vi "Acquisition and Generation Engine.vi"() -> ()   [LabVIEW 2015]
uses:
  Controls/Wave Generator Control.ctl
  Controls/WT1800 Readings.ctl
  Controls/WT1800 Measurements.ctl
  Controls/DSA Readings.ctl
  Controls/DSA Measurements.ctl
  Controls/WT1800 Functions.ctl
  Controls/DSA Functions.ctl
  Controls/Settings Control.ctl
  Controls/Channel Configuration Cluster.ctl
  Controls/Channel Configuration List.ctl
  Controls/Gain Averages.ctl
  Controls/Channel Configuration Cluster High Current.ctl
  Controls/Gain Array.ctl
panel:
  out "Supply Low":bool
  out "Test Time":dbl format="%<%H:%M:%S>t"
  in  "Tab Control":enum32{"Numeric", "Graph", "GUI Controls"}(tab)
  out "DSA Measurements":T1 {"Vrms" format="%.3f"; "Vdc" format="%.3f"; "Vpk+" format="%.3f"; "Vpk-" format="%.3f"; "Vpkpk" format="%.3f"}
  out "WT1800 Measurements":T3 {"Vrms" format="%.3f"; "Irms" format="%.3f"; "Power" format="%.3f"; "Vpkpk" format="%.3f"; "Ipkpk" format="%.3f"}
  out "DSA Averages":T1 {"Vrms" format="%.3f"; "Vdc" format="%.3f"; "Vpk+" format="%.3f"; "Vpk-" format="%.3f"; "Vpkpk" format="%.3f"}
  out "WT1800 Functions":T5
  out "WT1800 Averages":T3 {"Vrms" format="%.3f"; "Irms" format="%.3f"; "Power" format="%.3f"; "Vpkpk" format="%.3f"; "Ipkpk" format="%.3f"}
  out "DSA Functions":T6
  out "Graph":dbl[][](graph)
  in  "Wave Generator Cluster":T7={"Signal Amplitude [Vrms]"=0.1, "Signal Type"=0, "Frequency Range [Hz]"={"start"=150.0, "stop"=0.0}, "Waveform Duration [Seconds]"=10.0} {"Signal Type" items=["Sine", "Linear Chirp", "Log Chirp", "Pink Noise", "Periodic Random Noise", "Uniform White Noise", "Gaussian White Noise", "11db4816 Wave File"]}
  in  "Settings Cluster":T8={"Supply Voltage [Vdc]"=14.4, "Max Supply Current [Idc]"=50.0, "Settling Delay"=10.0, "Temp Criteria"=0.0, "Voltage Steps [Vrms]"=[0.25, 0.5, 1.0, 1.95, 3.0, 3.9, 5.5], "User Notes"="", "Config Wave File Path"=path "", "Config Voltage [Vrms]"=0.0, "Channel Configuration List"={"Channel Configuration Cluster"={"Input"=enum."---", "Enable"=FALSE, "User Notes"="", "Voltage Range"=15.0, "Current Range"=2.5}, "Channel Configuration Cluster 2"={"Input"=enum."---", "Enable"=FALSE, "User Notes"="", "Voltage Range"=15.0, "Current Range"=2.5}, "Channel Configuration Cluster 3"={"Input"=enum."---", "Enable"=FALSE, "User Notes"="", "Voltage Range"=15.0, "Current Range"=2.5}, "Channel Configuration Cluster 4"={"Input"=enum."---", "Enable"=FALSE, "User Notes"="", "Voltage Range"=15.0, "Current Range"=2.5}, "Channel Configuration Cluster 5"={"Input"=enum."---", "Enable"=FALSE, "User Notes"="", "Voltage Range"=15.0, "Current Range"=2.5}, "Channel Configuration Cluster 6"={"Input"=enum."---", "Enable"=FALSE, "User Notes"="", "Voltage Range"=15.0, "Current Range"=2.5}, "Channel Configuration Cluster 7"={"Input"=enum."---", "Enable"=FALSE, "User Notes"="", "Voltage Range"=15.0, "Current Range"=2.5}, "Channel Configuration Cluster 8"={"Input"=enum."---", "Enable"=FALSE, "User Notes"="", "Voltage Range"=15.0, "Current Range"=2.5}, "Channel Configuration Cluster 9"={"Input"=enum."---", "Enable"=FALSE, "User Notes"="", "Voltage Range"=15.0, "Current Range"=2.5}, "Channel Configuration Cluster 10"={"Input"=enum."---", "Enable"=FALSE, "User Notes"="", "Voltage Range"=15.0, "Current Range"=25.0}, "Channel Configuration Cluster 11"={"Input"=enum."---", "Enable"=FALSE, "User Notes"="", "Voltage Range"=15.0, "Current Range"=25.0}, "Channel Configuration Cluster 12"={"Input"=enum."---", "Enable"=FALSE, "User Notes"="", "Voltage Range"=15.0, "Current Range"=25.0}, "Channel Configuration Cluster 13"={"Input"=enum."---", "Enable"=FALSE, "User Notes"="", "Voltage Range"=15.0, "Current Range"=25.0}, "Channel Configuration Cluster 14"={"Input"=enum."---", "Enable"=FALSE, "User Notes"="", "Voltage Range"=15.0, "Current Range"=25.0}, "Channel Configuration Cluster 15"={"Input"=enum."---", "Enable"=FALSE, "User Notes"="", "Voltage Range"=15.0, "Current Range"=25.0}, "Channel Configuration Cluster 16"={"Input"=enum."---", "Enable"=FALSE, "User Notes"="", "Voltage Range"=15.0, "Current Range"=25.0}, "Channel Configuration Cluster 17"={"Input"=enum."---", "Enable"=FALSE, "User Notes"="", "Voltage Range"=15.0, "Current Range"=25.0}}, "User Gains"={"Gain 1"=0.0, "Gain 2"=0.0, "Gain 3"=0.0, "Gain 4"=0.0, "Gain 5"=0.0, "Gain 6"=0.0}, "Gains"={"Gain 1"=0.0, "Gain 2"=0.0, "Gain 3"=0.0, "Gain 4"=0.0, "Gain 5"=0.0, "Gain 6"=0.0}, "Gain Array"={"Gain 1"=0.0, "Gain 2"=0.0, "Gain 3"=0.0, "Gain 4"=0.0, "Gain 5"=0.0, "Gain 6"=0.0, "Gain 7"=0.0, "Gain 8"=0.0, "Gain 9"=0.0, "Gain 10"=0.0, "Gain 11"=0.0, "Gain 12"=0.0, "Gain 13"=0.0, "Gain 14"=0.0, "Gain 15"=0.0, "Gain 16"=0.0, "Gain 17"=0.0}, "Wave File Path 1"=path "", "Wave File Path 2"=path "", "Wave File Path 3"=path "", "Wave File Path 4"=path "", "Range"=FALSE, "CF"=FALSE} {"Gain Array"."Gain 17" format="%.2f"; "Gain Array"."Gain 16" format="%.2f"; "Gain Array"."Gain 15" format="%.2f"; "Gain Array"."Gain 14" format="%.2f"; "Gain Array"."Gain 13" format="%.2f"; "Gain Array"."Gain 12" format="%.2f"; "Gain Array"."Gain 11" format="%.2f"; "Gain Array"."Gain 10" format="%.2f"; "Gain Array"."Gain 9" format="%.2f"; "Gain Array"."Gain 8" format="%.2f"; "Gain Array"."Gain 7" format="%.2f"; "Gain Array"."Gain 6" format="%.2f"; "Gain Array"."Gain 5" format="%.2f"; "Gain Array"."Gain 4" format="%.2f"; "Gain Array"."Gain 3" format="%.2f"; "Gain Array"."Gain 2" format="%.2f"; "Gain Array"."Gain 1" format="%.2f"; "Gains"."Gain 6" format="%.2f"; "Gains"."Gain 5" format="%.2f"; "Gains"."Gain 4" format="%.2f"; "Gains"."Gain 3" format="%.2f"; "Gains"."Gain 2" format="%.2f"; "Gains"."Gain 1" format="%.2f"; "User Gains"."Gain 6" format="%.2f"; "User Gains"."Gain 5" format="%.2f"; "User Gains"."Gain 4" format="%.2f"; "User Gains"."Gain 3" format="%.2f"; "User Gains"."Gain 2" format="%.2f"; "User Gains"."Gain 1" format="%.2f"; "Channel Configuration List"."Channel Configuration Cluster 17"."Current Range" items=["1 <500m>"=0.5, "2 <1>"=1.0, "5 <2.5>"=2.5, "10 <5>"=5.0, "20 <10>"=10.0, "50 <25>"=25.0]; "Channel Configuration List"."Channel Configuration Cluster 17"."Voltage Range" items=["1.5 <0.75>"=0.75, "3 <1.5>"=1.5, "6 <3>"=3.0, "10 <5>"=5.0, "15 <7.5>"=7.5, "30 <15>"=15.0, "60 <30>"=30.0, "100 <50>"=50.0, "150 <75>"=75.0, "300 <150>"=150.0, "600 <300>"=300.0, "1000 <500>"=500.0]; "Channel Configuration List"."Channel Configuration Cluster 16"."Current Range" items=["1 <500m>"=0.5, "2 <1>"=1.0, "5 <2.5>"=2.5, "10 <5>"=5.0, "20 <10>"=10.0, "50 <25>"=25.0]; "Channel Configuration List"."Channel Configuration Cluster 16"."Voltage Range" items=["1.5 <0.75>"=0.75, "3 <1.5>"=1.5, "6 <3>"=3.0, "10 <5>"=5.0, "15 <7.5>"=7.5, "30 <15>"=15.0, "60 <30>"=30.0, "100 <50>"=50.0, "150 <75>"=75.0, "300 <150>"=150.0, "600 <300>"=300.0, "1000 <500>"=500.0]; "Channel Configuration List"."Channel Configuration Cluster 15"."Current Range" items=["1 <500m>"=0.5, "2 <1>"=1.0, "5 <2.5>"=2.5, "10 <5>"=5.0, "20 <10>"=10.0, "50 <25>"=25.0]; "Channel Configuration List"."Channel Configuration Cluster 15"."Voltage Range" items=["1.5 <0.75>"=0.75, "3 <1.5>"=1.5, "6 <3>"=3.0, "10 <5>"=5.0, "15 <7.5>"=7.5, "30 <15>"=15.0, "60 <30>"=30.0, "100 <50>"=50.0, "150 <75>"=75.0, "300 <150>"=150.0, "600 <300>"=300.0, "1000 <500>"=500.0]; "Channel Configuration List"."Channel Configuration Cluster 14"."Current Range" items=["1 <500m>"=0.5, "2 <1>"=1.0, "5 <2.5>"=2.5, "10 <5>"=5.0, "20 <10>"=10.0, "50 <25>"=25.0]; "Channel Configuration List"."Channel Configuration Cluster 14"."Voltage Range" items=["1.5 <0.75>"=0.75, "3 <1.5>"=1.5, "6 <3>"=3.0, "10 <5>"=5.0, "15 <7.5>"=7.5, "30 <15>"=15.0, "60 <30>"=30.0, "100 <50>"=50.0, "150 <75>"=75.0, "300 <150>"=150.0, "600 <300>"=300.0, "1000 <500>"=500.0]; "Channel Configuration List"."Channel Configuration Cluster 13"."Current Range" items=["1 <500m>"=0.5, "2 <1>"=1.0, "5 <2.5>"=2.5, "10 <5>"=5.0, "20 <10>"=10.0, "50 <25>"=25.0]; "Channel Configuration List"."Channel Configuration Cluster 13"."Voltage Range" items=["1.5 <0.75>"=0.75, "3 <1.5>"=1.5, "6 <3>"=3.0, "10 <5>"=5.0, "15 <7.5>"=7.5, "30 <15>"=15.0, "60 <30>"=30.0, "100 <50>"=50.0, "150 <75>"=75.0, "300 <150>"=150.0, "600 <300>"=300.0, "1000 <500>"=500.0]; "Channel Configuration List"."Channel Configuration Cluster 12"."Current Range" items=["1 <500m>"=0.5, "2 <1>"=1.0, "5 <2.5>"=2.5, "10 <5>"=5.0, "20 <10>"=10.0, "50 <25>"=25.0]; "Channel Configuration List"."Channel Configuration Cluster 12"."Voltage Range" items=["1.5 <0.75>"=0.75, "3 <1.5>"=1.5, "6 <3>"=3.0, "10 <5>"=5.0, "15 <7.5>"=7.5, "30 <15>"=15.0, "60 <30>"=30.0, "100 <50>"=50.0, "150 <75>"=75.0, "300 <150>"=150.0, "600 <300>"=300.0, "1000 <500>"=500.0]; "Channel Configuration List"."Channel Configuration Cluster 11"."Current Range" items=["1 <500m>"=0.5, "2 <1>"=1.0, "5 <2.5>"=2.5, "10 <5>"=5.0, "20 <10>"=10.0, "50 <25>"=25.0]; "Channel Configuration List"."Channel Configuration Cluster 11"."Voltage Range" items=["1.5 <0.75>"=0.75, "3 <1.5>"=1.5, "6 <3>"=3.0, "10 <5>"=5.0, "15 <7.5>"=7.5, "30 <15>"=15.0, "60 <30>"=30.0, "100 <50>"=50.0, "150 <75>"=75.0, "300 <150>"=150.0, "600 <300>"=300.0, "1000 <500>"=500.0]; "Channel Configuration List"."Channel Configuration Cluster 10"."Current Range" items=["1 <500m>"=0.5, "2 <1>"=1.0, "5 <2.5>"=2.5, "10 <5>"=5.0, "20 <10>"=10.0, "50 <25>"=25.0]; "Channel Configuration List"."Channel Configuration Cluster 10"."Voltage Range" items=["1.5 <0.75>"=0.75, "3 <1.5>"=1.5, "6 <3>"=3.0, "10 <5>"=5.0, "15 <7.5>"=7.5, "30 <15>"=15.0, "60 <30>"=30.0, "100 <50>"=50.0, "150 <75>"=75.0, "300 <150>"=150.0, "600 <300>"=300.0, "1000 <500>"=500.0]; "Channel Configuration List"."Channel Configuration Cluster 9"."Voltage Range" items=["1.5 <0.75>"=0.75, "3 <1.5>"=1.5, "6 <3>"=3.0, "10 <5>"=5.0, "15 <7.5>"=7.5, "30 <15>"=15.0, "60 <30>"=30.0, "100 <50>"=50.0, "150 <75>"=75.0, "300 <150>"=150.0, "600 <300>"=300.0, "1000 <500>"=500.0]; "Channel Configuration List"."Channel Configuration Cluster 9"."Current Range" items=["10m <5m>"=0.005, "20m <10m>"=0.01, "50m <25m>"=0.025, "100m <50m>"=0.05, "200m <100m>"=0.1, "500m <250m>"=0.25, "1 <500m>"=0.5, "2 <1>"=1.0, "5 <2.5>"=2.5]; "Channel Configuration List"."Channel Configuration Cluster 8"."Voltage Range" items=["1.5 <0.75>"=0.75, "3 <1.5>"=1.5, "6 <3>"=3.0, "10 <5>"=5.0, "15 <7.5>"=7.5, "30 <15>"=15.0, "60 <30>"=30.0, "100 <50>"=50.0, "150 <75>"=75.0, "300 <150>"=150.0, "600 <300>"=300.0, "1000 <500>"=500.0]; "Channel Configuration List"."Channel Configuration Cluster 8"."Current Range" items=["10m <5m>"=0.005, "20m <10m>"=0.01, "50m <25m>"=0.025, "100m <50m>"=0.05, "200m <100m>"=0.1, "500m <250m>"=0.25, "1 <500m>"=0.5, "2 <1>"=1.0, "5 <2.5>"=2.5]; "Channel Configuration List"."Channel Configuration Cluster 7"."Voltage Range" items=["1.5 <0.75>"=0.75, "3 <1.5>"=1.5, "6 <3>"=3.0, "10 <5>"=5.0, "15 <7.5>"=7.5, "30 <15>"=15.0, "60 <30>"=30.0, "100 <50>"=50.0, "150 <75>"=75.0, "300 <150>"=150.0, "600 <300>"=300.0, "1000 <500>"=500.0]; "Channel Configuration List"."Channel Configuration Cluster 7"."Current Range" items=["10m <5m>"=0.005, "20m <10m>"=0.01, "50m <25m>"=0.025, "100m <50m>"=0.05, "200m <100m>"=0.1, "500m <250m>"=0.25, "1 <500m>"=0.5, "2 <1>"=1.0, "5 <2.5>"=2.5]; "Channel Configuration List"."Channel Configuration Cluster 6"."Voltage Range" items=["1.5 <0.75>"=0.75, "3 <1.5>"=1.5, "6 <3>"=3.0, "10 <5>"=5.0, "15 <7.5>"=7.5, "30 <15>"=15.0, "60 <30>"=30.0, "100 <50>"=50.0, "150 <75>"=75.0, "300 <150>"=150.0, "600 <300>"=300.0, "1000 <500>"=500.0]; "Channel Configuration List"."Channel Configuration Cluster 6"."Current Range" items=["10m <5m>"=0.005, "20m <10m>"=0.01, "50m <25m>"=0.025, "100m <50m>"=0.05, "200m <100m>"=0.1, "500m <250m>"=0.25, "1 <500m>"=0.5, "2 <1>"=1.0, "5 <2.5>"=2.5]; "Channel Configuration List"."Channel Configuration Cluster 5"."Voltage Range" items=["1.5 <0.75>"=0.75, "3 <1.5>"=1.5, "6 <3>"=3.0, "10 <5>"=5.0, "15 <7.5>"=7.5, "30 <15>"=15.0, "60 <30>"=30.0, "100 <50>"=50.0, "150 <75>"=75.0, "300 <150>"=150.0, "600 <300>"=300.0, "1000 <500>"=500.0]; "Channel Configuration List"."Channel Configuration Cluster 5"."Current Range" items=["10m <5m>"=0.005, "20m <10m>"=0.01, "50m <25m>"=0.025, "100m <50m>"=0.05, "200m <100m>"=0.1, "500m <250m>"=0.25, "1 <500m>"=0.5, "2 <1>"=1.0, "5 <2.5>"=2.5]; "Channel Configuration List"."Channel Configuration Cluster 4"."Voltage Range" items=["1.5 <0.75>"=0.75, "3 <1.5>"=1.5, "6 <3>"=3.0, "10 <5>"=5.0, "15 <7.5>"=7.5, "30 <15>"=15.0, "60 <30>"=30.0, "100 <50>"=50.0, "150 <75>"=75.0, "300 <150>"=150.0, "600 <300>"=300.0, "1000 <500>"=500.0]; "Channel Configuration List"."Channel Configuration Cluster 4"."Current Range" items=["10m <5m>"=0.005, "20m <10m>"=0.01, "50m <25m>"=0.025, "100m <50m>"=0.05, "200m <100m>"=0.1, "500m <250m>"=0.25, "1 <500m>"=0.5, "2 <1>"=1.0, "5 <2.5>"=2.5]; "Channel Configuration List"."Channel Configuration Cluster 3"."Voltage Range" items=["1.5 <0.75>"=0.75, "3 <1.5>"=1.5, "6 <3>"=3.0, "10 <5>"=5.0, "15 <7.5>"=7.5, "30 <15>"=15.0, "60 <30>"=30.0, "100 <50>"=50.0, "150 <75>"=75.0, "300 <150>"=150.0, "600 <300>"=300.0, "1000 <500>"=500.0]; "Channel Configuration List"."Channel Configuration Cluster 3"."Current Range" items=["10m <5m>"=0.005, "20m <10m>"=0.01, "50m <25m>"=0.025, "100m <50m>"=0.05, "200m <100m>"=0.1, "500m <250m>"=0.25, "1 <500m>"=0.5, "2 <1>"=1.0, "5 <2.5>"=2.5]; "Channel Configuration List"."Channel Configuration Cluster 2"."Voltage Range" items=["1.5 <0.75>"=0.75, "3 <1.5>"=1.5, "6 <3>"=3.0, "10 <5>"=5.0, "15 <7.5>"=7.5, "30 <15>"=15.0, "60 <30>"=30.0, "100 <50>"=50.0, "150 <75>"=75.0, "300 <150>"=150.0, "600 <300>"=300.0, "1000 <500>"=500.0]; "Channel Configuration List"."Channel Configuration Cluster 2"."Current Range" items=["10m <5m>"=0.005, "20m <10m>"=0.01, "50m <25m>"=0.025, "100m <50m>"=0.05, "200m <100m>"=0.1, "500m <250m>"=0.25, "1 <500m>"=0.5, "2 <1>"=1.0, "5 <2.5>"=2.5]; "Channel Configuration List"."Channel Configuration Cluster"."Voltage Range" items=["1.5 <0.75>"=0.75, "3 <1.5>"=1.5, "6 <3>"=3.0, "10 <5>"=5.0, "15 <7.5>"=7.5, "30 <15>"=15.0, "60 <30>"=30.0, "100 <50>"=50.0, "150 <75>"=75.0, "300 <150>"=150.0, "600 <300>"=300.0, "1000 <500>"=500.0]; "Channel Configuration List"."Channel Configuration Cluster"."Current Range" items=["10m <5m>"=0.005, "20m <10m>"=0.01, "50m <25m>"=0.025, "100m <50m>"=0.05, "200m <100m>"=0.1, "500m <250m>"=0.25, "1 <500m>"=0.5, "2 <1>"=1.0, "5 <2.5>"=2.5]; "Settling Delay" min=0.0}
  out "Error Out":errorcluster
  in  "Error In":errorcluster
  out "Test Delay":dbl format="%<%H:%M:%S>t"
  out "Voltage Step":dbl format="%.3g"
  out "Scan Rate":dbl format="%.3g"
  in  "Abort":bool
  # "Ch1"
  # "Ch2"
  # "Ch3"
  # "Ch4"
  # "Ch5"
  # "Ch6"
  # "Ch7"
  # "Ch8"
  # "Ch9"
  # "Ch10"
  # "Ch11"
  # "Ch12"
  # "Ch13"
  # "Ch14"
  # "Ch15"
  # "Ch16"
  # "Ch17"
  # "PS Ch18"
  # "DSA Ch1"
  # "DSA Ch2"
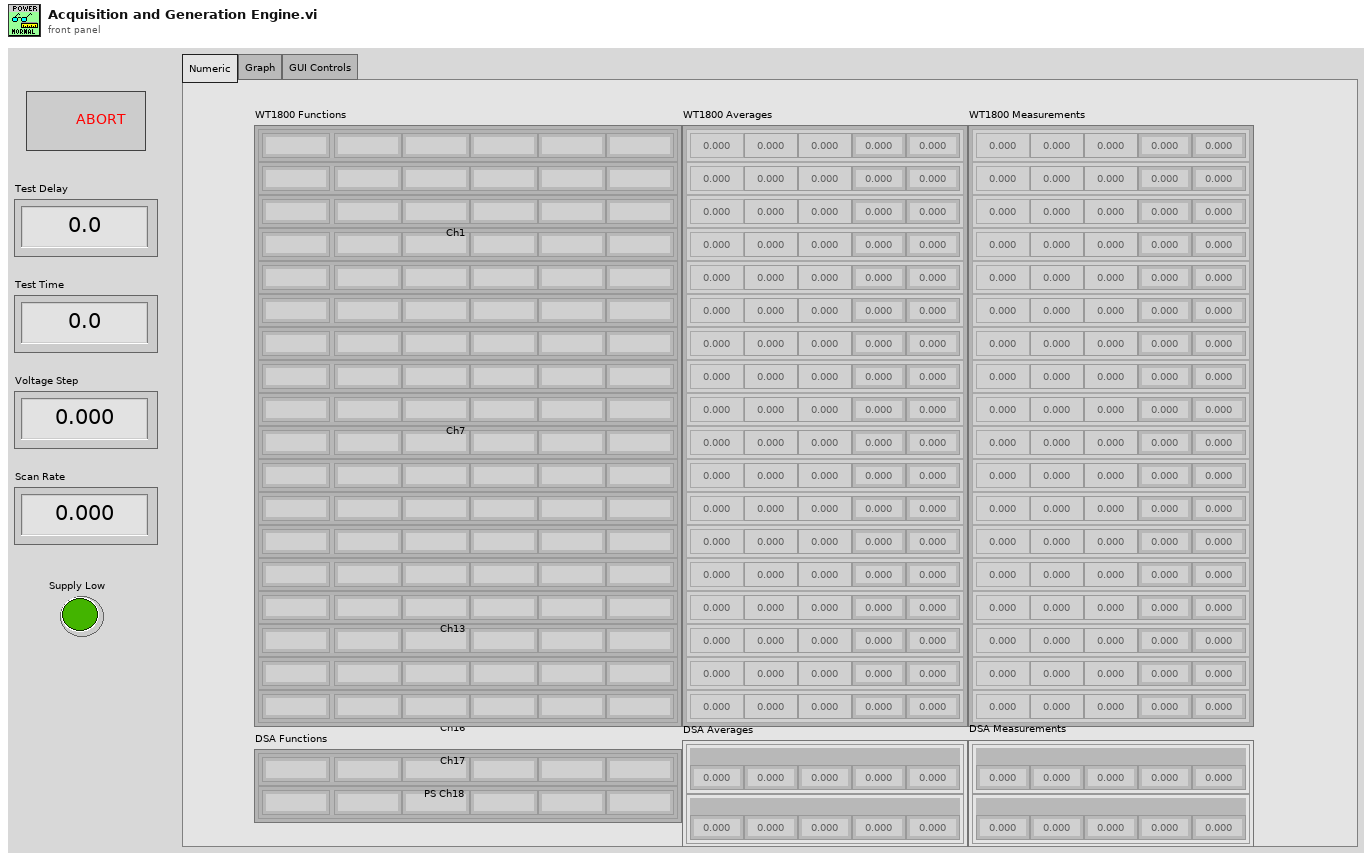
[diagram p1: front panel]
types:
  T1 = typedef "DSA Measurements.ctl" = T2[]
  T2 = typedef "DSA Readings.ctl" = cluster{"Vrms":dbl, "Vdc":dbl, "Vpk+":dbl, "Vpk-":dbl, "Vpkpk":dbl}
  T3 = typedef "WT1800 Measurements.ctl" = T4[]
  T4 = typedef "WT1800 Readings.ctl" = cluster{"Vrms":dbl, "Irms":dbl, "Power":dbl, "Vpkpk":dbl, "Ipkpk":dbl}
  T5 = typedef "WT1800 Functions.ctl" = cluster{"Channel":string, "Vrms":string, "Power":string, "Vpkpk":string, "Ipkpk":string, "Vpkpk":string}[]
  T6 = typedef "DSA Functions.ctl" = cluster{"Channel":string, "Vrms":string, "Vdc":string, "Vpk+":string, "Vpk-":string, "Vpkpk":string}[]
  T7 = typedef "Wave Generator Control.ctl" = cluster{"Signal Amplitude [Vrms]":dbl, "Signal Type":u16, "Frequency Range [Hz]":cluster{"start":dbl, "stop":dbl}, "Waveform Duration [Seconds]":dbl}
  T8 = typedef "Settings Control.ctl" = cluster{"Supply Voltage [Vdc]":dbl, "Max Supply Current [Idc]":dbl, "Settling Delay":dbl, "Temp Criteria":dbl, "Voltage Steps [Vrms]":dbl[], "User Notes":string, "Config Wave File Path":path, "Config Voltage [Vrms]":dbl, "Channel Configuration List":T9, "User Gains":T12, "Gains":T12, "Gain Array":T13, "Wave File Path 1":path, "Wave File Path 2":path, "Wave File Path 3":path, "Wave File Path 4":path, "Range":bool, "CF":bool}
  T9 = typedef "Channel Configuration List.ctl" = cluster{"Channel Configuration Cluster":T10, "Channel Configuration Cluster 2":T10, "Channel Configuration Cluster 3":T10, "Channel Configuration Cluster 4":T10, "Channel Configuration Cluster 5":T10, "Channel Configuration Cluster 6":T10, "Channel Configuration Cluster 7":T10, "Channel Configuration Cluster 8":T10, "Channel Configuration Cluster 9":T10, "Channel Configuration Cluster 10":T11, "Channel Configuration Cluster 11":T11, "Channel Configuration Cluster 12":T11, "Channel Configuration Cluster 13":T11, "Channel Configuration Cluster 14":T11, "Channel Configuration Cluster 15":T11, "Channel Configuration Cluster 16":T11, "Channel Configuration Cluster 17":T11}
  T10 = typedef "Channel Configuration Cluster.ctl" = cluster{"Input":enum16{"---", "1", "1 AVG", "2", "2 AVG", "3", "3 AVG", "4", "4 AVG"}, "Enable":bool, "User Notes":string, "Voltage Range":dbl, "Current Range":dbl}
  T11 = typedef "Channel Configuration Cluster High Current.ctl" = cluster{"Input":enum16{"---", "1", "1 AVG", "2", "2 AVG", "3", "3 AVG", "4", "4 AVG"}, "Enable":bool, "User Notes":string, "Voltage Range":dbl, "Current Range":dbl}
  T12 = typedef "Gain Averages.ctl" = cluster{"Gain 1":dbl, "Gain 2":dbl, "Gain 3":dbl, "Gain 4":dbl, "Gain 5":dbl, "Gain 6":dbl}
  T13 = typedef "Gain Array.ctl" = cluster{"Gain 1":dbl, "Gain 2":dbl, "Gain 3":dbl, "Gain 4":dbl, "Gain 5":dbl, "Gain 6":dbl, "Gain 7":dbl, "Gain 8":dbl, "Gain 9":dbl, "Gain 10":dbl, "Gain 11":dbl, "Gain 12":dbl, "Gain 13":dbl, "Gain 14":dbl, "Gain 15":dbl, "Gain 16":dbl, "Gain 17":dbl}
  T14 = enum32{"Home", "Channel Configuration", "Power Test"}
  T15 = cluster{"AI Task ID In":refnum<k21>[], "AO Task ID In":refnum<k21>[]}
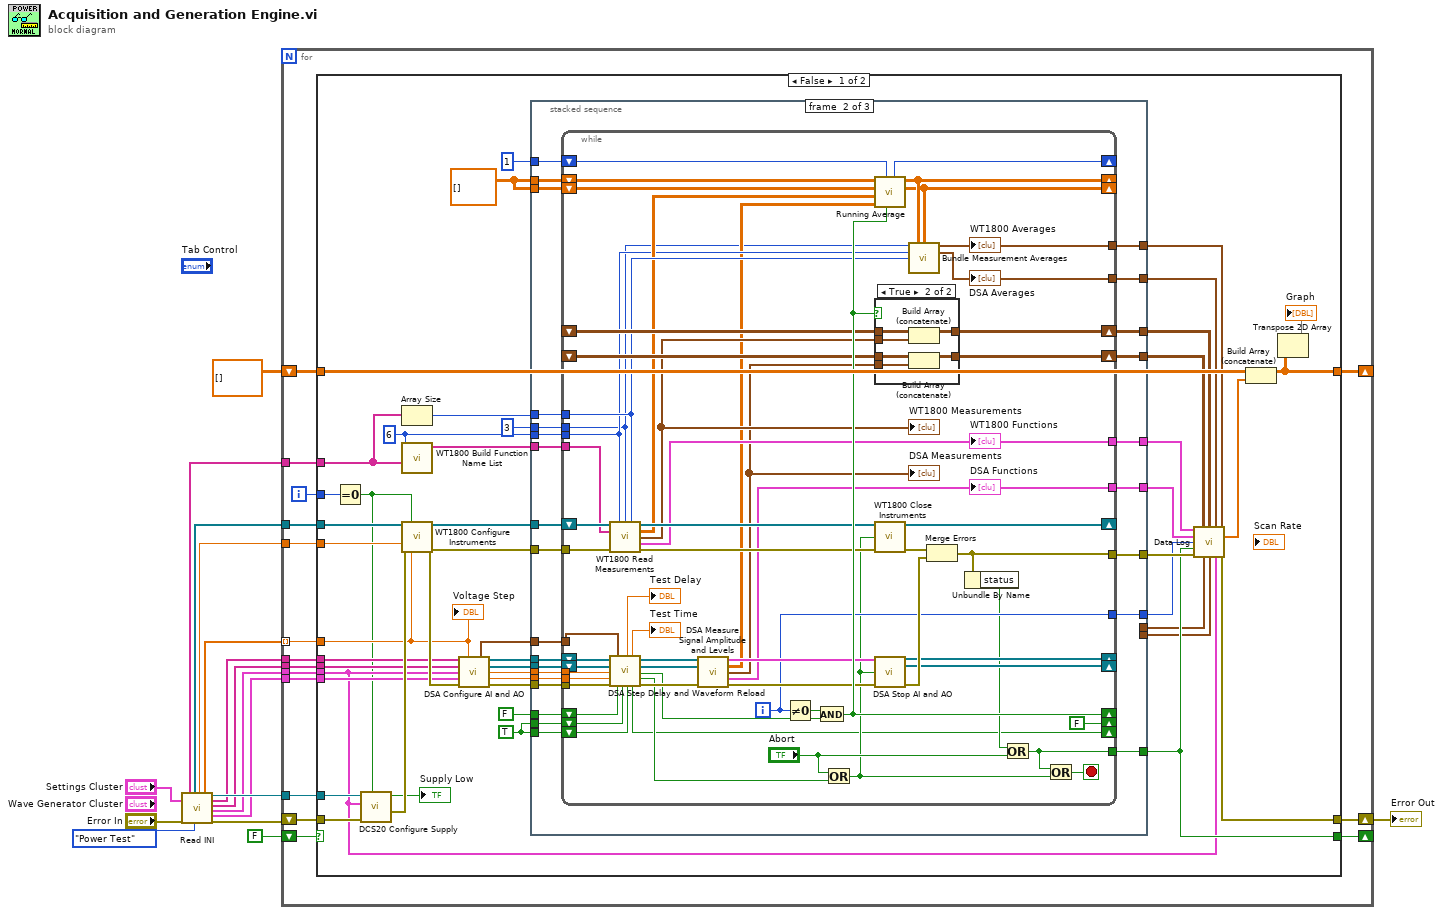
[diagram p0: block diagram]
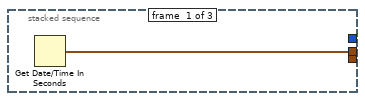
[diagram p2: hidden frame]
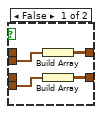
[diagram p3: hidden frame]
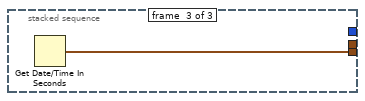
[diagram p4: hidden frame]
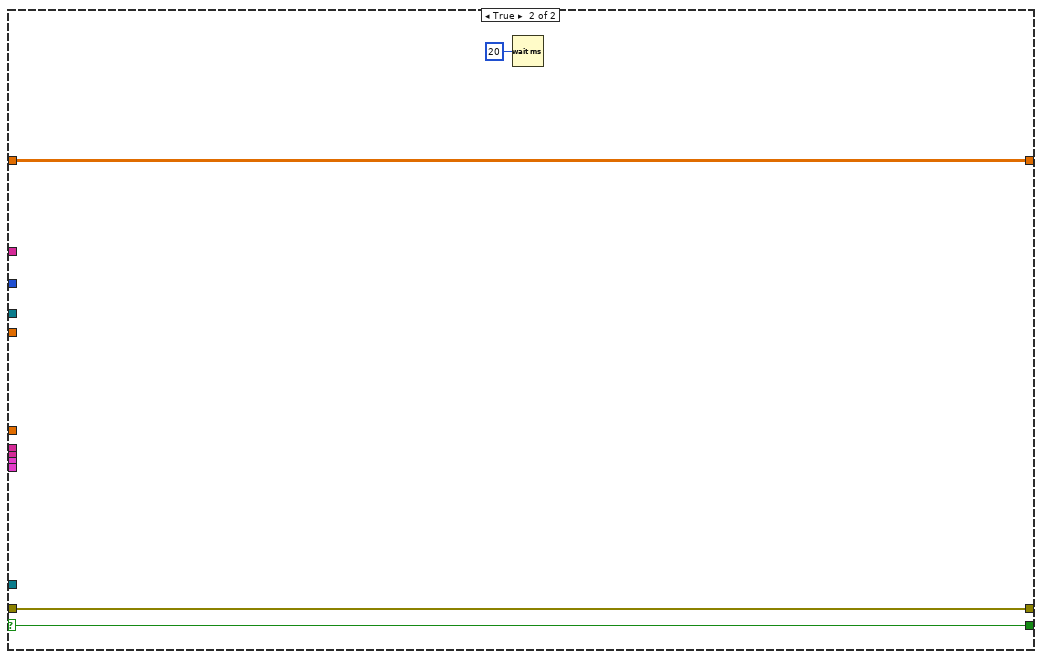
[diagram p5: hidden frame]
diagram:
  n1 = call "Read INI.vi"("Settings Cluster In"="Settings Cluster", "Error In"="Error In", "Command"=T14."Power Test" ("Tab Control")) -> ("Functions To Retreive"=w12:string[], "WT1800 Instruments"=w11:refnum<visa-resource-name>[], "Update Rate [Seconds]"=w10:dbl, "Voltage Steps [Vrms]"=w9:dbl[], "DC Power Supply"=w16:refnum<visa-resource-name>, "DSA Input Channels"=w6:tag[], "DSA Output Channels"=w5:tag[], "Settings Cluster Out"=w3:T8, "Wave Generator Cluster Out"=w4:T7, "Error Out"=w8:errorcluster)  [unwired: 4 in, 3 out]
  n2 = for {
    tunnel: w6 -> [w31]
    tunnel: w5 -> [w30]
    tunnel: w10 -> [w29]
    tunnel: w11 -> [w32]
    tunnel: w9 -> [w24] mode=indexing
    tunnel: w12 -> [w28]
    shift-right: [w27] -> w14
    shift-left: w8 -> [w23]
    tunnel: w16 -> [w26]
    shift-right: [w22] -> _
    shift-left: FALSE -> [w21]
    shift-right: [w20] -> _
    shift-left: dbl[][] [] ("Graph") -> [w19]
    tunnel: w3 -> [w18]
    tunnel: w4 -> [w17]
    i -> [w25]
    n3 = case shown="False" w21 {
      selector: w21 -> [_ w180]
      tunnel: w32 -> [w72 _]
      tunnel: w31 -> [w65 _]
      tunnel: w30 -> [w64 _]
      tunnel: w29 -> [w62 _]
      tunnel: w28 -> [w61 _]
      tunnel: [w60 w181] -> w27
      tunnel: w23 -> [w75 w181]
      tunnel: w26 -> [w58 _]
      tunnel: w25 -> [w57 _]
      tunnel: w24 -> [w37 _]
      tunnel: [w47 w180] -> w22
      tunnel: [w45 w179] -> w20
      tunnel: w19 -> [w78 w179]
      tunnel: w18 -> [w35 _]
      tunnel: w17 -> [w36 _]
      frame False {
        w42 = TRUE ("Reset Delay Clock")
        w69 = 6 ("Number of Elements")
        w43 = dbl[][] []
        n4 = Equal To 0?(x=w57) -> (x = 0?=w34:bool)
        n5 = call "DCS20 Configure Supply.vi"("Initialize"=w34, "Error In"=w75, "Settings Cluster"=w35, "DC Power Supply In"=w58) -> ("Errors Out"=w77:errorcluster[], "Supply Voltage Lower Than Expected"=→"Supply Low":bool)  [unwired: 6 in]
        n6 = Array Size(array=w61) -> (size(s)=w67:i32)
        n7 = call "WT1800 Build Function Name List.vi"("Functions To Retreive"=w61, "Number of Channels"=w69) -> ("Array out"=w66:string[])  [unwired: 9 in]
        n8 = call "WT1800 Configure Instruments.vi"("WT1800 Instruments In"=w72, "Check EQ"=w34, "Update Rate (50ms)"=w62, "Error In"=w77, "Voltage Step"=w37) -> ("WT1800 Instruments Out"=w71:refnum<visa-resource-name>[], "Errors Out"=w76:errorcluster[])  [unwired: 9 in]
        n9 = call "DSA Configure AI and AO.vi"("Input  Physical Channel"=w65, "Voltage Step"=w37, "Output Physical Channel"=w64, "Settings Cluster"=w35, "Wave Generator Cluster"=w36, "Errors In"=w76) -> ("Waveform"=w56:waveform(dbl)[], "AI Task ID Out"=w74:refnum<k21>[], "AO Task ID Out"=w73:refnum<k21>[], "Waveform Duration"=w55:dbl, "Step Delay"=w54:dbl, "Errors Out"=w53:errorcluster[])  [unwired: 3 in, 1 out]
        n10 = stacked-sequence {
          tunnel: w74 -> [_ w106 _]
          tunnel: w43 -> [_ w105 _]
          tunnel: w73 -> [_ w104 _]
          tunnel: w71 -> [_ w103 _]
          tunnel: 1 ("Iteration Count") -> [_ w102 _]
          tunnel: w69 -> [_ w101 _]
          tunnel: 3 ("Channel Group") -> [_ w100 _]
          tunnel: w67 -> [_ w99 _]
          tunnel: w66 -> [_ w98 _]
          tunnel: FALSE ("Time has Elapsed In") -> [_ w97 _]
          tunnel: [_ w96 _] -> w59
          tunnel: w76 -> [_ w95 _]
          tunnel: w56 -> [_ w94 _]
          tunnel: [_ _ w177] -> w38
          tunnel: w55 -> [_ w93 _]
          tunnel: w54 -> [_ w92 _]
          tunnel: w42 -> [_ w91 _]
          tunnel: w42 -> [_ w90 _]
          tunnel: [_ w89 _] -> w48
          tunnel: [_ w88 _] -> w47
          tunnel: w53 -> [_ w87 _]
          tunnel: [_ w86 _] -> w52
          tunnel: [_ w85 _] -> w51
          tunnel: [_ w84 _] -> w50
          tunnel: [_ w83 _] -> w49
          tunnel: [w79 _ _] -> w39
          tunnel: [_ w82 _] -> w40
          tunnel: [_ w81 _] -> w41
          tunnel: w43 -> [_ w80 _]
          frame #0 {
            n11 = Get Date/Time In Seconds() -> (seconds since 1Jan1904=w79:timestamp)
          }
          frame #1 {
            n12 = while {
              tunnel: w101 -> [w131]
              tunnel: w99 -> [w146]
              shift-right: [w149] -> _
              shift-left: w105 -> [w152]
              shift-right: [w147] -> _
              shift-left: w80 -> [w148]
              tunnel: w100 -> [w107]
              tunnel: w98 -> [w142]
              tunnel: w87 -> [w150]
              shift-right: [w132] -> _
              shift-left: w102 -> [w130]
              shift-right: [w166] -> _
              shift-left: w97 -> [w123]
              tunnel: w95 -> [w144]
              tunnel: w94 -> [w141]
              tunnel: [w138] -> w96
              shift-right: [w156] -> _
              shift-left: w106 -> [w136]
              shift-right: [w155] -> _
              shift-left: w104 -> [w137]
              shift-right: [w134] -> _
              shift-left: w103 -> [w153]
              shift-right: [w133] -> w85
              shift-left: _ -> [w158]
              tunnel: [w113] -> w84
              shift-right: [FALSE ("Reset Delay Clock")] -> _
              shift-left: w91 -> [w119]
              tunnel: [w154] -> w89
              tunnel: [w126] -> w88
              tunnel: w93 -> [w125]
              tunnel: w92 -> [w124]
              shift-right: [w116] -> _
              shift-left: w90 -> [w117]
              tunnel: [w114] -> w83
              shift-right: [w115] -> w86
              shift-left: _ -> [w157]
              tunnel: [w160] -> w82
              tunnel: [w159] -> w81
              i -> [w154]
              stop <- w127 stop-if-true
              n13 = call "WT1800 Read Measurements.vi"("WT1800 Instruments In"=w153, "WT1800 Channels per Instrument"=w131, "WT1800 Channel Group"=w107, "Number of Functions"=w146, "Desired Functions"=w142, "Errors In"=w144) -> ("WT1800 Instruments Out"=w165:refnum<visa-resource-name>[], 6:"WT1800 Measurements"=w145:dbl[][], 8:"WT1800 Measurements"=w110:T3, "WT1800 Functions"=w159:T5, "Errors Out"=w164:errorcluster[])  [unwired: 5 in]
              "WT1800 Measurements" <- w110
              "WT1800 Functions" <- w159
              n14 = call "DSA Step Delay and Waveform Reload.vi"("AI Task ID In"=w136, "AO Task ID In"=w137, "Waveform Duration"=w125, "Step Delay"=w124, "Errors In"=w150, "AO Waveform"=w141, "Step Delay Time has Elapsed In"=w123, "Reset Delay Clock In"=w119, "Reset Test Clock In"=w117) -> ("Step Delay Count Down"=→"Test Delay":dbl, "Test Count Down"=→"Test Time":dbl, "Reset Test Clock Out"=w116:bool, "AI Task ID Out"=w140:refnum<k21>[], "AO Task ID Out"=w139:refnum<k21>[], "Step Delay Time has Elapsed Out"=w112:bool, "Test Time has Elapsed Out"=w120:bool, "Errors Out"=w143:errorcluster[])  [unwired: 2 in, 1 out]
              n15 = call "DSA Measure Signal Amplitude and Levels.vi"("AI Task ID In"=w140, "AO Task ID In"=w139, "Errors In"=w143) -> ("Task ID Cluster"=w163:T15, "DSA Measurements Array"=w109:dbl[][], "DSA Measurements"=w108:T1, "DSA Functions"=w160:T6, "Errors Out"=w162:errorcluster[])  [unwired: 8 in]
              "DSA Measurements" <- w108
              "DSA Functions" <- w160
              n16 = Not Equal To 0?(x=w154) -> (x != 0?=w111:bool)
              n17 = And(x=w111, y=w112) -> (x .and. y?=w166:bool)
              n18 = Or(x="Abort", y=w120) -> (x .or. y?=w128:bool)
              n19 = call "Running Average.vi"("Load Data"=w166, "Iteration Count In"=w130, "DSA Measurements In"=w109, "WT1800 Measurements In"=w145, "DSA Averages In"=w148, "WT1800 Averages In"=w152) -> ("DSA Averages Out"=w147:dbl[][], "WT1800 Averages Out"=w149:dbl[][], "Iteration Count Out"=w132:i32)  [unwired: 3 in]
              n20 = case shown="True" w166 {
                tunnel: w110 -> [w169 w174]
                tunnel: w158 -> [_ w176]
                tunnel: [w170 w175] -> w133
                tunnel: w108 -> [w168 w172]
                tunnel: [w167 w171] -> w115
                tunnel: w157 -> [_ w173]
                frame False {
                  n21 = Build Array(w169) -> (w170:T4[][])
                  n22 = Build Array(w168) -> (w167:T2[][])
                }
                frame True {
                  n23 = Build Array (concatenate)(w176, w174) -> (w175:T4[][])
                  n24 = Build Array (concatenate)(w173, w172) -> (w171:T2[][])
                }
              }
              n25 = call "WT1800 Close Instruments.vi"("WT1800 Instruments In"=w165, "Buffer Complete In"=w128, "Errors In"=w164) -> ("WT1800 Instruments Out"=w134:refnum<visa-resource-name>[], "Errors Out"=w135:errorcluster[])  [unwired: 10 in, 1 out]
              n26 = call "DSA Stop AI and AO.vi"("Task ID Cluster"=w163, "Buffer Complete"=w128, "Errors In"=w162) -> ("AI Task ID Out"=w156:refnum<k21>[], "AO Task ID Out"=w155:refnum<k21>[], "Errors Out"=w161:errorcluster[])  [unwired: 10 in]
              n27 = call "Bundle Measurement Averages.vi"("WT1800 Channel Group"=w107, "WT1800 Measurements"=w149, "DSA Measurements"=w147, "WT1800 Channels per Instrument"=w131, "Number of Functions"=w146) -> ("WT1800 Averages"=w114:T3, "DSA Averages"=w113:T1)  [unwired: 8 in, 1 out]
              "WT1800 Averages" <- w114
              "DSA Averages" <- w113
              n28 = Merge Errors(w135, w161) -> (w138:errorcluster)
              n29 = Unbundle By Name ("名前でバンドル解除")(w138) -> ("status"=w151:bool)
              n30 = Or(x=w151, y="Abort") -> (x .or. y?=w126:bool)
              n31 = Or(x=w126, y=w128) -> (x .or. y?=w127:bool)
            }
          }
          frame #2 {
            n32 = Get Date/Time In Seconds() -> (seconds since 1Jan1904=w177:timestamp)
          }
        }
        n33 = call "Data Log.vi"("WT1800 Functions"=w41, "DSA Measurements"=w52, "WT1800 Measurements"=w51, "DSA Averages"=w50, "WT1800 Averages"=w49, "DSA Functions"=w40, "Iteration Count"=w48, "Error or Abort"=w47, "error in"=w59, "Initial Time Stamp"=w39, "Final Time Stamp"=w38, "Settings Cluster"=w35) -> ("Average Power"=w46:dbl[], "error out"=w60:errorcluster)  [unwired: 2 out]
        n34 = Build Array (concatenate)(w78, w46) -> (w45:dbl[][])
        n35 = Transpose 2D Array(2D array=w45) -> (transposed array=→"Graph":dbl[][])
        "Voltage Step" <- w37
      }
      frame True {
        n36 = Wait (ms)(milliseconds to wait=u32 20) -> ()  [unwired: 1 out]
      }
    }
  }
  "Error Out" <- w14
